vi "Serial_Set(SCI_read).vi"(2 "baud rate (9600)":u32=115200 caption="보 전송속도(9600)", 4 "Port":refnum<visa-resource-name>="COM4" caption="VISA 리소스 이름") -> (0 "Error Out":errorcluster caption="에러 출력", 1 "VISA out":refnum<visa-resource-name>)   [LabVIEW 2010]
uses:
  <vilib>/Instr/_visa.llb/VISA Flush IO Buffer Mask.ctl
  <vilib>/Instr/_visa.llb/VISA Configure Serial Port (Instr).vi
panel:
  out "Commend Count":u32
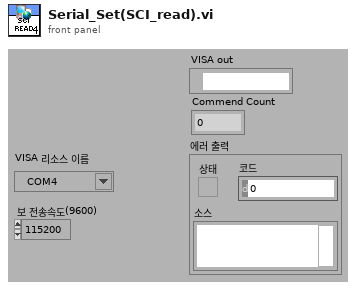
[diagram p1: front panel]
types:
  T1 = typedef "VISA Flush IO Buffer Mask.ctl" = u16
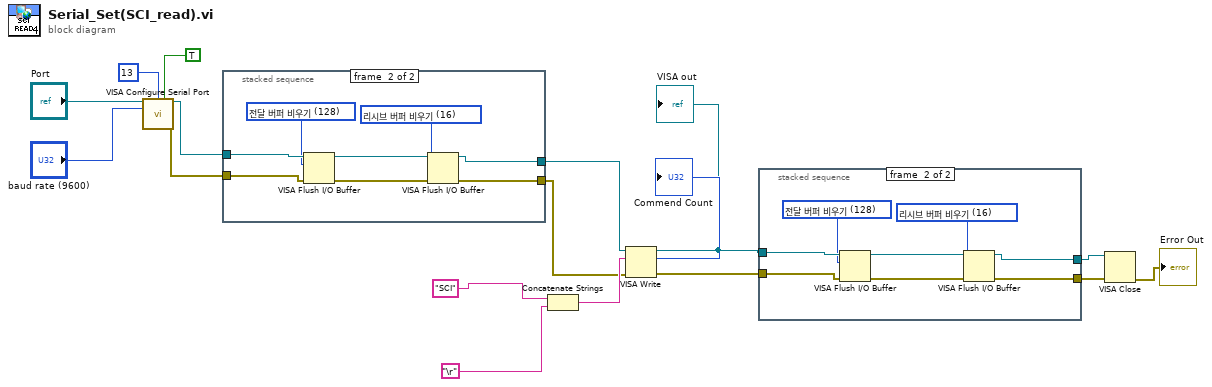
[diagram p0: block diagram]
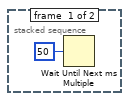
[diagram p2: hidden frame]
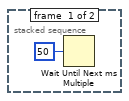
[diagram p3: hidden frame]
diagram:
  n1 = call-poly "VISA Configure Serial Port"("VISA resource name"="Port", "termination char\n(0xA = '\\n' = LF)"=i16 13 ("termination char\n(0xA = '\\n' = LF)"), "Enable Termination\nChar (T)"=TRUE ("Enable Termination\nChar (T)"), "baud rate (9600)"="baud rate (9600)") -> ("VISA resource name out"=w10:refnum<visa-resource-name>, "error out"=w9:errorcluster)  [unwired: 10 in]
  n2 = stacked-sequence {
    tunnel: w10 -> [_ w26]
    tunnel: w9 -> [_ w25]
    tunnel: [_ w21] -> w8
    tunnel: [_ w20] -> w7
    frame #0 {
      n3 = Wait Until Next ms Multiple(millisecond multiple=u32 50 ("ms 배수")) -> ()  [unwired: 1 out]
    }
    frame #1 {
      w19 = T1 16 items=["리시브 버퍼 비우기"=16, "전달 버퍼 디바이스에 쓰기"=32, "리시브 버퍼 비우기(I/O 없음)"=64, "전달 버퍼 비우기"=128] ("Mask")
      w24 = T1 128 items=["리시브 버퍼 비우기"=16, "전달 버퍼 디바이스에 쓰기"=32, "리시브 버퍼 비우기(I/O 없음)"=64, "전달 버퍼 비우기"=128] ("Mask")
      n4 = VISA Flush I/O Buffer(VISA resource name=w26, mask (16)=w24, error in (no error)=w25) -> (VISA resource name out=w23:refnum<visa-resource-name>, error out=w22:errorcluster)
      n5 = VISA Flush I/O Buffer(VISA resource name=w23, mask (16)=w19, error in (no error)=w22) -> (VISA resource name out=w21:refnum<visa-resource-name>, error out=w20:errorcluster)
    }
  }
  n6 = Concatenate Strings("SCI", "\r") -> (w16:string)
  n7 = VISA Write(VISA resource name=w8, write buffer=w16, error in (no error)=w7) -> (VISA resource name out=w4:refnum<visa-resource-name>, return count=→"Commend Count":u32, error out=w3:errorcluster)
  "VISA out" <- w4
  n8 = stacked-sequence {
    tunnel: w4 -> [_ w35]
    tunnel: w3 -> [_ w34]
    tunnel: [_ w30] -> w5
    tunnel: [_ w29] -> w6
    frame #0 {
      n9 = Wait Until Next ms Multiple(millisecond multiple=u32 50 ("ms 배수")) -> ()  [unwired: 1 out]
    }
    frame #1 {
      w28 = T1 16 items=["리시브 버퍼 비우기"=16, "전달 버퍼 디바이스에 쓰기"=32, "리시브 버퍼 비우기(I/O 없음)"=64, "전달 버퍼 비우기"=128] ("Mask")
      w33 = T1 128 items=["리시브 버퍼 비우기"=16, "전달 버퍼 디바이스에 쓰기"=32, "리시브 버퍼 비우기(I/O 없음)"=64, "전달 버퍼 비우기"=128] ("Mask")
      n10 = VISA Flush I/O Buffer(VISA resource name=w35, mask (16)=w33, error in (no error)=w34) -> (VISA resource name out=w32:refnum<visa-resource-name>, error out=w31:errorcluster)
      n11 = VISA Flush I/O Buffer(VISA resource name=w32, mask (16)=w28, error in (no error)=w31) -> (VISA resource name out=w30:refnum<visa-resource-name>, error out=w29:errorcluster)
    }
  }
  n12 = VISA Close(VISA resource name=w5, error in (no error)=w6) -> (error out=→"Error Out":errorcluster)
